vi "OrderExecuted.generated.vi"(11 "buffer.in":u64[](array[numeric])=[0, 0, 0, 0, 0, 0, 0, 0, 0]) -> (3 "OrderBook.Command":T1)   [LabVIEW 2020]
doc: "Cboe PITCH Order Executed (0x23) and Order Executed at Price/Size (0x24) -> orderbook.command: type OrderExecuted or OrderExecutedAtPrice, orderId, executed.qty, remaining.qty and price (0x24 only), nanoseconds, Edit."
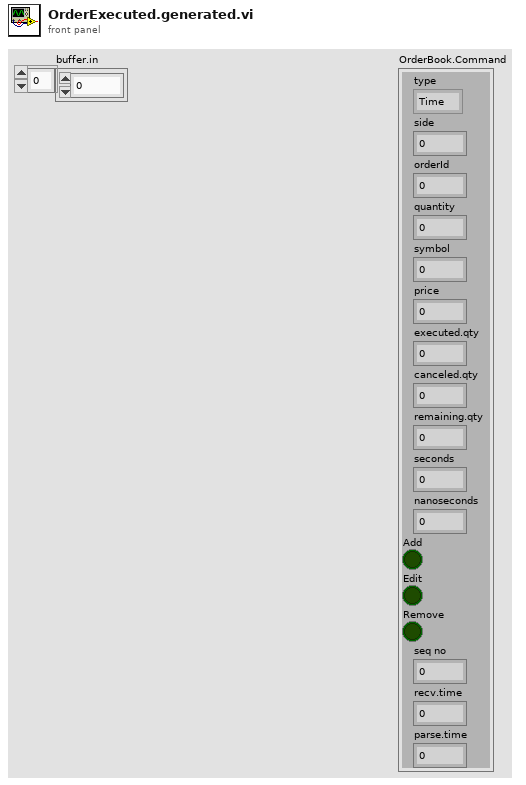
[diagram p1: front panel]
types:
  T1 = cluster{"type":enum8{"Time", "AddOrder", "OrderExecuted", "OrderExecutedAtPrice", "ReduceSize", "ModifyOrder", "DeleteOrder", "Get.Everything", "Get.All.Orders", "Get.Top"}, "side":u8, "orderId ":u64, "quantity":u32, "symbol":u64, "price":u64, "executed.qty":u32, "canceled.qty":u32, "remaining.qty":u32, "seconds":u64, "nanoseconds":u64, "Add":bool, "Edit":bool, "Remove":bool, "seq no":u32, "recv.time":u64, "parse.time":u64}
  T2 = enum8{"Time", "AddOrder", "OrderExecuted", "OrderExecutedAtPrice", "ReduceSize", "ModifyOrder", "DeleteOrder", "Get.Everything", "Get.All.Orders", "Get.Top"}
  T3 = cluster{"type":enum8{"Time", "AddOrder", "OrderExecuted", "OrderExecutedAtPrice", "ReduceSize", "ModifyOrder", "DeleteOrder", "Get.Everything", "Get.All.Orders", "Get.Top"}, "side":u8, "orderId ":u64, "quantity":u32, "symbol":u64, "price":u64, u32, "canceled.qty":u32, "remaining_qty":u32, "seconds":u64, "nanoseconds":u64, "Add":bool, "Edit":bool, "Remove":bool, "seq no":u32, "recv.time":u64, "parse.time":u64}
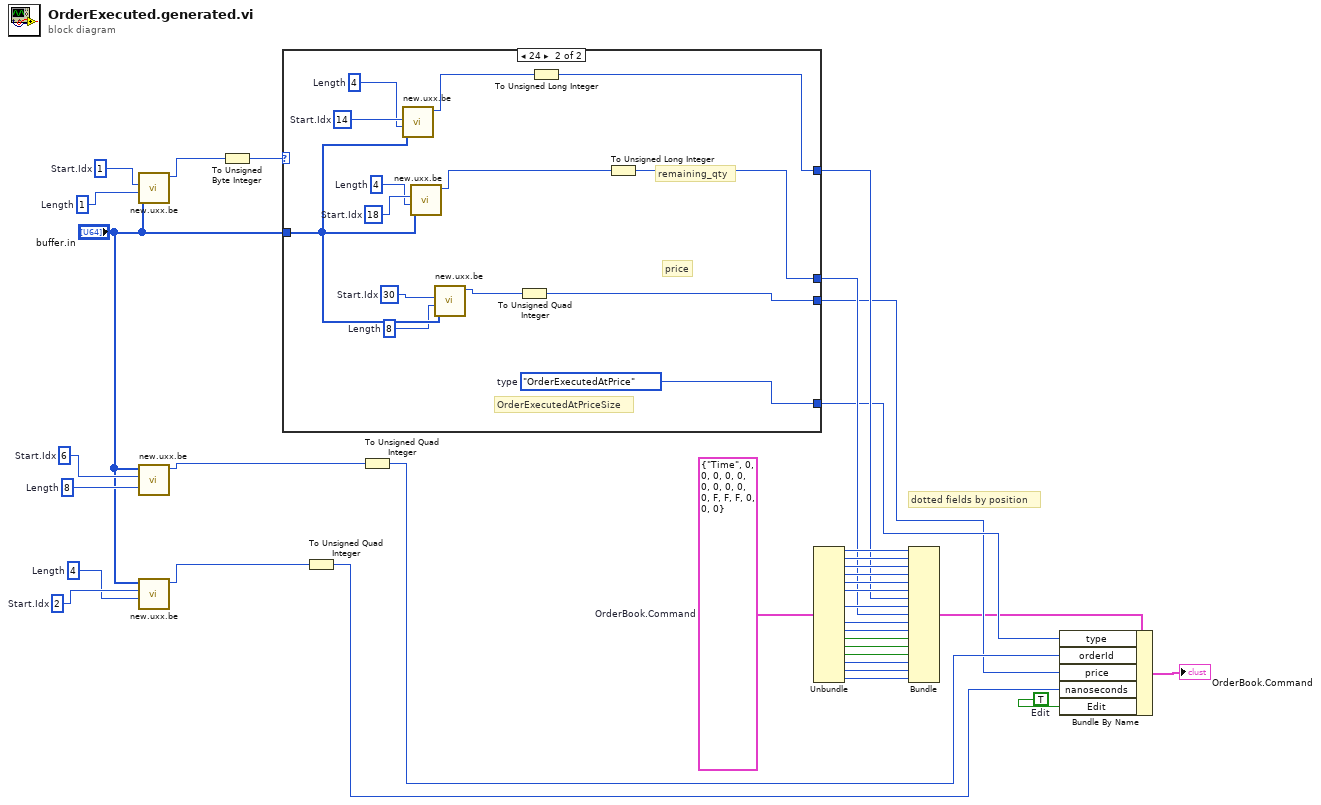
[diagram p0: block diagram]
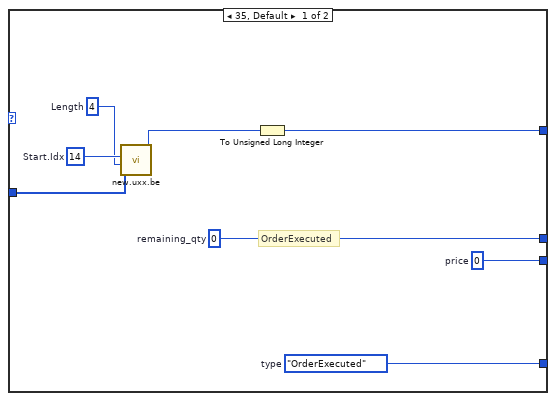
[diagram p2: hidden frame]
diagram:
  w29 = u8 8  # Length
  w30 = u8 6  # Start.Idx
  w32 = u8 4  # Length
  w33 = u8 2  # Start.Idx
  w35 = u8 1  # Length
  w36 = u8 1  # Start.Idx
  w3 = TRUE  # Edit
  w25 = T1 {"type"=enum."Time", "side"=0, "orderId "=0, "quantity"=0, "symbol"=0, "price"=0, "executed.qty"=0, "canceled.qty"=0, "remaining.qty"=0, "seconds"=0, "nanoseconds"=0, "Add"=FALSE, "Edit"=FALSE, "Remove"=FALSE, "seq no"=0, "recv.time"=0, "parse.time"=0}  # OrderBook.Command
  # "dotted fields by position"
  n1 = call "new.uxx.be.vi"("buffer (U64)"="buffer.in", "Start.Idx"=w36, "Length"=w35) -> ("Out.Value U64"=w34:u64)  [unwired: 7 in]
  n2 = call "new.uxx.be.vi"("buffer (U64)"="buffer.in", "Start.Idx"=w30, "Length"=w29) -> ("Out.Value U64"=w28:u64)  [unwired: 7 in]
  n3 = call "new.uxx.be.vi"("buffer (U64)"="buffer.in", "Start.Idx"=w33, "Length"=w32) -> ("Out.Value U64"=w31:u64)  [unwired: 7 in]
  n4 = To Unsigned Byte Integer(number=w34) -> (unsigned 8bit integer=w26:u8)
  n5 = case shown="24" w26 {
    tunnel: "buffer.in" -> [w44 w52]
    tunnel: [w40 w48] -> w7
    tunnel: [w39 w47] -> w18
    tunnel: [w38 w46] -> w16
    tunnel: [w37 w45] -> w5
    frame 35, Default {
      w37 = u64 0  # price
      w38 = u32 0  # remaining_qty
      w42 = u8 4  # Length
      w43 = u8 14  # Start.Idx
      w40 = T2."OrderExecuted"  # type
      # "OrderExecuted"
      n6 = call "new.uxx.be.vi"("buffer (U64)"=w44, "Start.Idx"=w43, "Length"=w42) -> ("Out.Value U64"=w41:u64)  [unwired: 7 in]
      n7 = To Unsigned Long Integer(number=w41) -> (unsigned 32bit integer=w39:u32)
    }
    frame 36 {
      w50 = u8 8  # Length
      w51 = u8 30  # Start.Idx
      w54 = u8 4  # Length
      w55 = u8 18  # Start.Idx
      w57 = u8 4  # Length
      w58 = u8 14  # Start.Idx
      w48 = T2."OrderExecutedAtPrice"  # type
      # "price"
      # "remaining_qty"
      # "OrderExecutedAtPriceSize"
      n8 = call "new.uxx.be.vi"("buffer (U64)"=w52, "Start.Idx"=w58, "Length"=w57) -> ("Out.Value U64"=w56:u64)  [unwired: 7 in]
      n9 = call "new.uxx.be.vi"("buffer (U64)"=w52, "Start.Idx"=w55, "Length"=w54) -> ("Out.Value U64"=w53:u64)  [unwired: 7 in]
      n10 = call "new.uxx.be.vi"("buffer (U64)"=w52, "Start.Idx"=w51, "Length"=w50) -> ("Out.Value U64"=w49:u64)  [unwired: 7 in]
      n11 = To Unsigned Quad Integer(1:w49) -> (0:w45:u64)
      n12 = To Unsigned Long Integer(number=w56) -> (unsigned 32bit integer=w47:u32)
      n13 = To Unsigned Long Integer(number=w53) -> (unsigned 32bit integer=w46:u32)
    }
  }
  n14 = To Unsigned Quad Integer(1:w31) -> (0:w4:u64)
  n15 = To Unsigned Quad Integer(1:w28) -> (0:w6:u64)
  n16 = Unbundle(w25) -> ("type"=w24:T2, "side"=w23:u8, "orderId"=w22:u64, "quantity"=w21:u32, "symbol"=w20:u64, "price"=w19:u64, "canceled.qty"=w17:u32, "seconds"=w15:u64, "nanoseconds"=w14:u64, "Add"=w13:bool, "Edit"=w12:bool, "Remove"=w11:bool, "seq no"=w10:u32, "recv.time"=w9:u64, "parse.time"=w8:u64)  [unwired: 2 out]
  n17 = Bundle("type"=w24, "side"=w23, "orderId"=w22, "quantity"=w21, "symbol"=w20, "price"=w19, w18, "canceled.qty"=w17, "remaining_qty"=w16, "seconds"=w15, "nanoseconds"=w14, "Add"=w13, "Edit"=w12, "Remove"=w11, "seq no"=w10, "recv.time"=w9, "parse.time"=w8) -> (w2:T3)  [unwired: 1 in]
  n18 = Bundle By Name(cluster=w2, "type"=w7, "orderId"=w6, "price"=w5, "nanoseconds"=w4, "Edit"=w3) -> (→"OrderBook.Command":T3)
